vi "saveUserAnd SystemConfigFiles.vi"(10 "controls":T1 {"allValues"."safetyLimits"."channelLimits"."channelID" items=["time", "gearbox", "compressor bearing", "shaft bearing", "oil outlet", "inlet 1", "inlet 2", "outlet 1", "outlet 2", "inlet pressure", "outlet pressure", "plenum pressure", "Motor speed", "new V-cone DP", "Motor power", "Accelerometer", "Hotwire 1", "oil pressure", "butterfly valve position", "ball valve position", "Legacy speed", "Torque speed", "pulsator encoder", "v-cone upstream 1", "v-cone upstream 2"]}) -> ()   [LabVIEW 2018]
uses:
  user interface/systemConfigUIControls.ctl
  type defs/channelLimitControl.ctl
  type defs/limitActions.ctl
  ICL-LabVIEW_General/data channels/parent class/Data Channel.lvclass
  RT/Type Defs/Message loop data.ctl
  RT/Type Defs/FPGA reference.ctl
  RT/Type Defs/RT Status.ctl
  RT/Type Defs/Analogue loop data.ctl
  RT/Communications loop/comms data.ctl
  RT/Type Defs/generic incident.ctl
  ICL-LabVIEW_General/Scanivalve API project/full interface/polymorphic/scanivalveConfig.ctl
  ICL-LabVIEW_General/Scanivalve API project/full interface/listS.ctl
  ICL-LabVIEW_General/Scanivalve API project/full interface/listC.ctl
  ICL-LabVIEW_General/Scanivalve API project/full interface/listSG.ctl
  ICL-LabVIEW_General/Scanivalve API project/full interface/chan1.ctl
  RT/Type Defs/Data processing loop data.ctl
  type defs/channelControl.ctl
  RT/Type Defs/channelScalingTypes.ctl
  RT/Type Defs/scalingMethods.ctl
  <vilib>/Utility/config.llb/Write Key (String).vi
  <vilib>/Utility/config.llb/Write Key (Path).vi
  <vilib>/Utility/config.llb/Write Key (U32).vi
  <vilib>/Utility/config.llb/Write Key (Boolean).vi
  <vilib>/Utility/config.llb/Write Key (Double).vi
  <vilib>/Utility/config.llb/NI_LVConfig.lvlib
  ICL-LabVIEW_General/data channels/data channels.lvlib
  ICL-LabVIEW_General/Scanivalve API project/Scanivalve API.lvlib
panel:
  out "error out":errorcluster
  out "unwritten keys":string[](array[string])
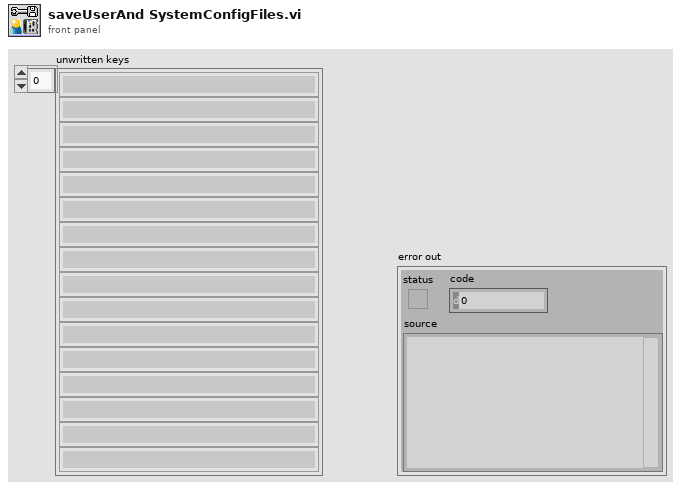
[diagram p1: front panel]
types:
  T1 = typedef "systemConfigUIControls.ctl" = cluster{"allControls":cluster{"feedbackChannels":cluster{"butterfly":refnum<vi>, "ball":refnum<vi>, "massflow":refnum<vi>, "pressureRatio":refnum<vi>, "airP":refnum<vi>, "water":refnum<vi>, "oilP":refnum<vi>, "speed":refnum<vi>}, "controlChannels":cluster{"butterflyControl":refnum<vi>, "ballControl":refnum<vi>, "speedControl":refnum<vi>}, "channelLimits":refnum<vi>, "pulsatorIP":string}, "allValues":cluster{"feedback":cluster{"butterfly":u16, "ball":u16, "massflow":u16, "pressureRatio":u16, "airP":u16, "water":u16, "oilP":u16, "speed":u16}, "paths":cluster{"channelConfig":path, "systemConfig":path, "incidentLogfile":path, "startFolder":path, "customVI":path}, "RT":cluster{"RTIP":string, "errorReaderName":string, "errorWriterName":string, "errorBufferSize":u16, "commandWriterName":string, "commandReaderName":string, "commandBufferSize":u16, "dataBufferSize":u16, "dataReaderName":string, "dataWriterName":string, "dataBufferLength":u16, "scanivalveIP":string, "scanPeriod":u16}, "controls":cluster{"butterflyControl":u16, "ballControl":u16, "speedControl":u16}, "safetyLimits":cluster{"channelLimits":T2[], "maxSpeed":u32}, "Howden":cluster{"howdenAir":bool, "howden%":dbl}}, "variables":cluster{"feedbackChannelIDs":u16[], "controlChannelIDs":u16[], "channelsArray":refnum<class "Data Channel.lvclass">[]}}
  T2 = typedef "channelLimitControl.ctl" = cluster{"channelID":u16, "Enabled":bool, "warnValue":dbl, "limitValue":dbl, "Invert":bool, "limitAction":T3}
  T3 = typedef "limitActions.ctl" = enum16{"stop", "shutdown", "ignore"}
  T4 = typedef "Message loop data.ctl" = cluster{"Parameters":cluster{"FPGA Ref":T5, "configID":u32, "activeChannels":cluster{"index":u16, "name":string}[]}, "Variables":cluster{"RT Status":T6, "watchdog":timestamp, "limitsEnabled":bool, "Interlocks":cluster{"gearboxOil":bool, "bearingOil":bool, "gearboxAir":bool}}}
  T5 = typedef "FPGA reference.ctl" = refnum<k20>
  T6 = typedef "RT Status.ctl" = cluster{"Comms loop":bool, "scheduler loop":bool, "data process loop":bool, "FIFO loop":bool, "Command Stream":bool, "Error Stream":bool, "FPGA FIFO":bool, "Data Stream":bool}
  T7 = typedef "Analogue loop data.ctl" = cluster{"Params":cluster{"FPGA ref":T5, "Total Channels":u32}, "Variables":cluster{"FIFO wait counter":u16, "FIFO read trigger":u32}}
  T8 = typedef "comms data.ctl" = cluster{"Parameters":cluster{"error writer name":string, "command reader name":string, "error buffer size":i32, "command buffer size":i32, "scanivalveIP":string, "scanivalvePeriod":u16}, "Variables":cluster{"listen schedule":u32, "incident buffer":T9[], "command stream":refnum<k21>, "error stream":refnum<k21>, "waiting for command stream connect":bool, "waiting for error stream connect":bool, "scanivalve connection":refnum<k5>, "scanivalveScheduleID":u32, "activeScanivalvePorts":i32[], "channelCount":i16}, "scanivalveConfig":T10}
  T9 = typedef "generic incident.ctl" = cluster{"timestamp":timestamp, "type":string, "Variant":variant}
  T10 = typedef "Scanivalve API.lvlib/scanivalveConfig.ctl" = cluster{"listS":T11, "listC":T12, "listSG":T13, "activeChannels":T14}
  T11 = typedef "Scanivalve API.lvlib/listS.ctl" = cluster{"period":u16, "ADtrig":bool, "ScanTrig":bool, "page":u16, "qpkts":u16}
  T12 = typedef "Scanivalve API.lvlib/listC.ctl" = cluster{"ZC":bool, "unitScan":string, "CvtUnit":dbl, "bin":bool, "EU":bool}
  T13 = typedef "Scanivalve API.lvlib/listSG.ctl" = cluster{"Avg1":u16, "FPS1":u16, "SGEnable1":bool}
  T14 = typedef "Scanivalve API.lvlib/chan1.ctl" = cluster{"Chan1":cluster{"101":bool, "102":bool, "103":bool, "104":bool, "109":bool, "110":bool, "111":bool, "112":bool, "201":bool, "202":bool, "203":bool, "204":bool, "209":bool, "210":bool, "211":bool, "212":bool, "301":bool, "302":bool, "303":bool, "304":bool, "309":bool, "310":bool, "311":bool, "312":bool, "401":bool, "402":bool, "403":bool, "404":bool, "409":bool, "410":bool, "411":bool, "412":bool}}
  T15 = typedef "Data processing loop data.ctl" = cluster{"Parameters":cluster{"FPGA Ref":T5, "data stream":cluster{"data writer name":string, "NS write buffer size":i32, "NS Buffer length":u32}, "FIFO Depth":u32, "Channel controls":cluster{"FIFO channel count":i32, "active indices":i16[], "active channels":i32, "channelScaling":T16[], "scanivalveCount":i32, "channels":refnum<class "Data Channel.lvclass">[]}, "safetyChannels":cluster{"oilP":u16, "airP":u16, "water":u16, "channelLimits":T2[]}, "speedChannel":i32, "maxSpeedLimit":dbl, "Torque":cluster{"fixedOffset":dbl, "filter":bool, "fallingEdge":bool, "swapEncoders":bool}}, "Variables":cluster{"Intermediary buffer":dbl[][], "buffer position":u32, "write loop counter":u16, "NS write trigger":u32, "NS Connection status":bool, "waiting for NS":bool, "labAmbient":cluster{"pressure":dbl, "temperature":dbl}, "scanivalvePorts":u16[], "scanivalvePressures":dbl[], "data stream":refnum<k21>, "activeChannelLimitIndex":u16[], "runningSpeedLimit":dbl, "speedChannelIndex":i32, "Interlocks":cluster{"gearboxOil":bool, "bearingOil":bool, "gearboxAir":bool}, "interlockChannels":cluster{"gearboxOil":i32, "bearingOil":i32, "air":i32}, "limitStates":cluster{"warn":bool, "alarm":bool}[]}}
  T16 = typedef "channelControl.ctl" = cluster{"index":u16, "active":bool, "channelType":T17, "module":u16, "terminal":u16, "channelName":string, "scalingMethod":T18, "scalingParameters":dbl[], "scaledUnits":string, "tempOffset":dbl}
  T17 = typedef "channelScalingTypes.ctl" = enum16{"calculation", "measurement", "scanivalve", "output", "digital"}
  T18 = typedef "scalingMethods.ctl" = enum16{"none", "linear", "thermocouple", "polynomial", "encoder", "RTD"}
  T19 = cluster{"Message":T4, "FIFO":T7, "Comms data":T8, "Data processor":T15}
  T20 = cluster{"total":cluster{"channels":u16, "FIFO":u16, "Scanivalve":u16, "Remote":u16, "Calculated":u16}, "active":cluster{"channels":u16, "FIFO":u16, "Scanivalve":u16, "Remote":u16, "Calculated":u16}}
  T21 = typedef "NI_LVConfig.lvlib/Config Data RefNum.ctl" = refnum<k1>
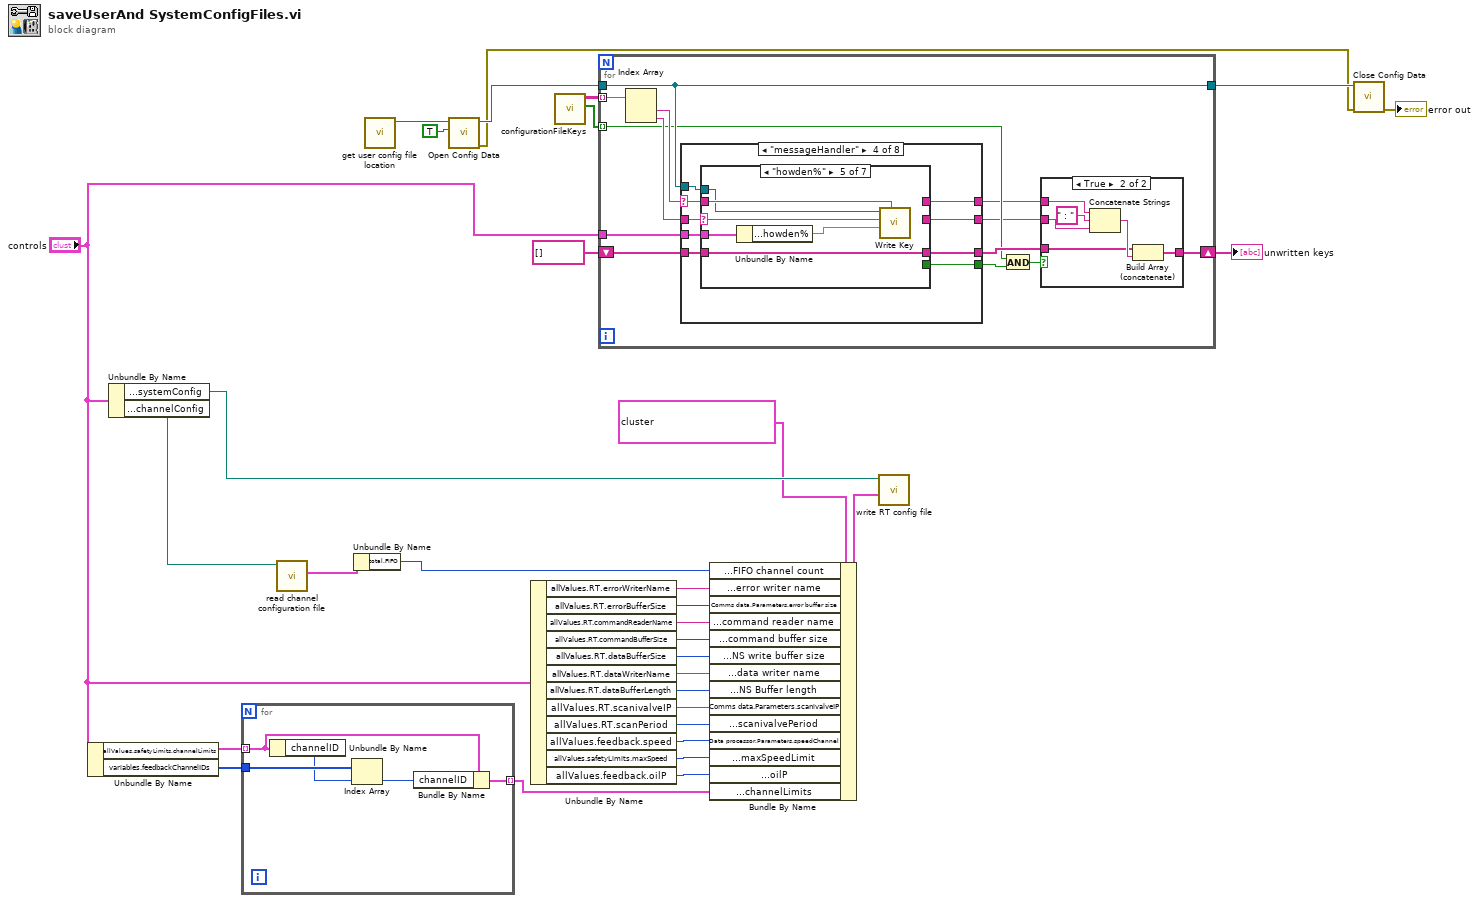
[diagram p0: block diagram]
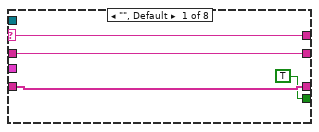
[diagram p3: hidden frame]
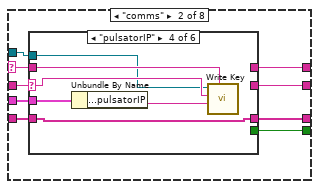
[diagram p4: hidden frame]
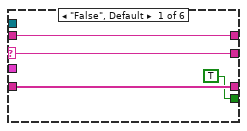
[diagram p5: hidden frame]
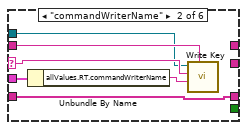
[diagram p6: hidden frame]
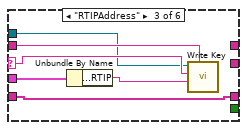
[diagram p7: hidden frame]
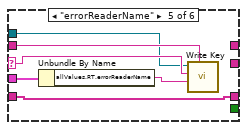
[diagram p8: hidden frame]
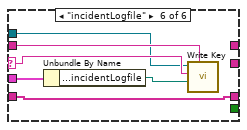
[diagram p9: hidden frame]
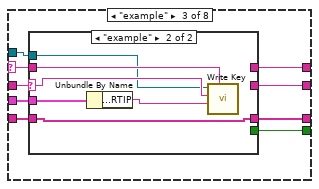
[diagram p10: hidden frame]
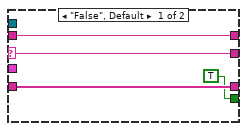
[diagram p11: hidden frame]
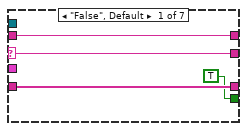
[diagram p12: hidden frame]
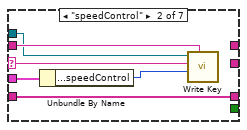
[diagram p13: hidden frame]
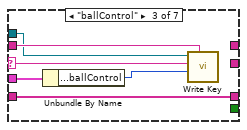
[diagram p14: hidden frame]
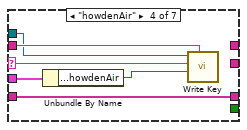
[diagram p15: hidden frame]
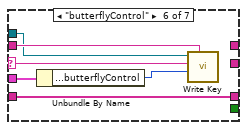
[diagram p16: hidden frame]
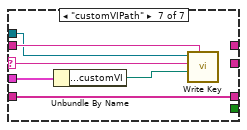
[diagram p17: hidden frame]
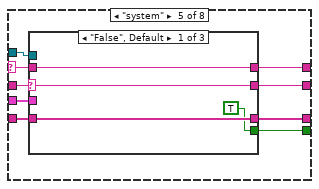
[diagram p18: hidden frame]
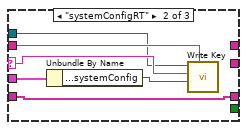
[diagram p19: hidden frame]
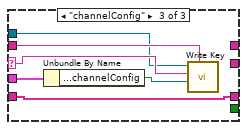
[diagram p20: hidden frame]
diagram:
  n1 = Unbundle By Name("controls") -> ("allValues.safetyLimits.channelLimits"=w10:T2[], "variables.feedbackChannelIDs"=w9:u16[])
  n2 = Unbundle By Name("controls") -> ("allValues.paths.systemConfig"=w22:path, "allValues.paths.channelConfig"=w5:path)
  n3 = for {
    tunnel: w10 -> [w34] mode=indexing
    tunnel: w9 -> [w37]
    tunnel: [w33] -> w1 mode=indexing
    n4 = Unbundle By Name(w34) -> ("channelID"=w36:u16)
    n5 = Index Array(array=w37, index=w36) -> (element=w35:u16)
    n6 = Bundle By Name(cluster=w34, "channelID"=w35) -> (w33:T2)
  }
  n7 = call "read channel configuration file.vi"("config file"=w5) -> ("counts"=w4:T20)  [unwired: 8 in, 2 out]
  n8 = Unbundle By Name(w4) -> ("total.FIFO"=w3:u16)
  n9 = call "get user config file location.vi"() -> ("userConfigPath"=w31:path)  [unwired: 11 in]
  n10 = call <vilib>:"Open Config Data.vi"("create file if necessary (T)"=TRUE, "configuration file path"=w31) -> ("error out"=w23:errorcluster, "refnum"=w30:T21)  [unwired: 7 in, 1 out]
  n11 = Unbundle By Name("controls") -> ("allValues.RT.errorWriterName"=w19:string, "allValues.RT.errorBufferSize"=w18:u16, "allValues.RT.commandReaderName"=w17:string, "allValues.RT.commandBufferSize"=w16:u16, "allValues.RT.dataBufferSize"=w15:u16, "allValues.RT.dataWriterName"=w14:string, "allValues.RT.dataBufferLength"=w13:u16, "allValues.RT.scanivalveIP"=w12:string, "allValues.RT.scanPeriod"=w11:u16, "allValues.feedback.speed"=w8:u16, "allValues.safetyLimits.maxSpeed"=w6:u32, "allValues.feedback.oilP"=w2:u16)
  n12 = call "configurationFileKeys.vi"() -> ("write user key?"=w25:bool[], "userConfigKeys"=w32:string[][])  [unwired: 9 in, 1 out]
  n13 = for {
    tunnel: "controls" -> [w46]
    tunnel: w32 -> [w50] mode=indexing
    tunnel: w30 -> [w47]
    tunnel: [w47] -> w29
    shift-right: [w43] -> w26
    shift-left: string[] [] -> [w45]
    tunnel: w25 -> [w41] mode=indexing
    n14 = Index Array(array=w50) -> (element #1=w49:string, element #2=w48:string)  [unwired: 2 in]
    n15 = case shown="\"messageHandler\"" w49 {
      selector: w49 -> [w61 w67 w110 w129 w178 w203 w252 w271]
      tunnel: w48 -> [w60 w70 w113 w132 w181 w206 w255 w274]
      tunnel: w47 -> [_ w69 w112 w131 w180 w205 w254 w273]
      tunnel: w46 -> [_ w68 w111 w130 w179 w204 w253 w272]
      tunnel: [w59 w66 w109 w128 w177 w202 w251 w270] -> w44
      tunnel: w45 -> [w59 w65 w108 w127 w176 w201 w250 w269]
      tunnel: [TRUE w62 w105 w124 w175 w198 w247 w266] -> w42
      tunnel: [w61 w64 w107 w126 w174 w200 w249 w268] -> w39
      tunnel: [w60 w63 w106 w125 w173 w199 w248 w267] -> w38
      frame "", Default {
      }
      frame "comms" {
        n16 = case shown="\"pulsatorIP\"" w70 {
          selector: w70 -> [w72 w79 w85 w91 w97 w103]
          tunnel: w69 -> [_ w78 w84 w90 w96 w102]
          tunnel: w68 -> [_ w77 w83 w89 w95 w101]
          tunnel: w67 -> [w73 w80 w86 w92 w98 w104]
          tunnel: [w74 w75 w81 w87 w93 w99] -> w66
          tunnel: w65 -> [w74 w75 w81 w87 w93 w99]
          tunnel: [w73 _ _ _ _ _] -> w64
          tunnel: [w72 _ _ _ _ _] -> w63
          tunnel: [TRUE _ _ _ _ _] -> w62
          frame "False", Default {
          }
          frame "commandWriterName" {
            n17 = Unbundle By Name(w77) -> ("allValues.RT.commandWriterName"=w76:string)
            n18 = call-poly <vilib>:"Write Key.vi"("section"=w80, "value"=w76, "key"=w79, "refnum"=w78) -> ()  [unwired: 5 in, 3 out]
          }
          frame "RTIPAddress" {
            n19 = Unbundle By Name(w83) -> ("allValues.RT.RTIP"=w82:string)
            n20 = call-poly <vilib>:"Write Key.vi"("section"=w86, "value"=w82, "key"=w85, "refnum"=w84) -> ()  [unwired: 5 in, 3 out]
          }
          frame "pulsatorIP" {
            n21 = Unbundle By Name(w89) -> ("allControls.pulsatorIP"=w88:string)
            n22 = call-poly <vilib>:"Write Key.vi"("section"=w92, "value"=w88, "key"=w91, "refnum"=w90) -> ()  [unwired: 5 in, 3 out]
          }
          frame "errorReaderName" {
            n23 = Unbundle By Name(w95) -> ("allValues.RT.errorReaderName"=w94:string)
            n24 = call-poly <vilib>:"Write Key.vi"("section"=w98, "value"=w94, "key"=w97, "refnum"=w96) -> ()  [unwired: 5 in, 3 out]
          }
          frame "incidentLogfile" {
            n25 = Unbundle By Name(w101) -> ("allValues.paths.incidentLogfile"=w100:path)
            n26 = call-poly <vilib>:"Write Key.vi"("section"=w104, "value"=w100, "key"=w103, "refnum"=w102) -> ()  [unwired: 5 in, 3 out]
          }
        }
      }
      frame "example" {
        n27 = case shown="\"example\"" w113 {
          selector: w113 -> [w115 w122]
          tunnel: w112 -> [_ w121]
          tunnel: w111 -> [_ w120]
          tunnel: w110 -> [w116 w123]
          tunnel: [w117 w118] -> w109
          tunnel: w108 -> [w117 w118]
          tunnel: [w116 _] -> w107
          tunnel: [w115 _] -> w106
          tunnel: [TRUE _] -> w105
          frame "False", Default {
          }
          frame "example" {
            n28 = Unbundle By Name(w120) -> ("allValues.RT.RTIP"=w119:string)
            n29 = call-poly <vilib>:"Write Key.vi"("section"=w123, "value"=w119, "key"=w122, "refnum"=w121) -> ()  [unwired: 5 in, 3 out]
          }
        }
      }
      frame "messageHandler" {
        n30 = case shown="\"howden%\"" w132 {
          selector: w132 -> [w134 w141 w147 w153 w159 w165 w171]
          tunnel: w131 -> [_ w140 w146 w152 w158 w164 w170]
          tunnel: w130 -> [_ w139 w145 w151 w157 w163 w169]
          tunnel: w129 -> [w135 w142 w148 w154 w160 w166 w172]
          tunnel: [w136 w137 w143 w149 w155 w161 w167] -> w128
          tunnel: w127 -> [w136 w137 w143 w149 w155 w161 w167]
          tunnel: [w135 _ _ _ _ _ _] -> w126
          tunnel: [w134 _ _ _ _ _ _] -> w125
          tunnel: [TRUE _ _ _ _ _ _] -> w124
          frame "False", Default {
          }
          frame "speedControl" {
            n31 = Unbundle By Name(w139) -> ("allValues.controls.speedControl"=w138:u16)
            n32 = call-poly <vilib>:"Write Key.vi"("section"=w142, "value"=w138, "key"=w141, "refnum"=w140) -> ()  [unwired: 5 in, 3 out]
          }
          frame "ballControl" {
            n33 = Unbundle By Name(w145) -> ("allValues.controls.ballControl"=w144:u16)
            n34 = call-poly <vilib>:"Write Key.vi"("section"=w148, "value"=w144, "key"=w147, "refnum"=w146) -> ()  [unwired: 5 in, 3 out]
          }
          frame "howdenAir" {
            n35 = Unbundle By Name(w151) -> ("allValues.Howden.howdenAir"=w150:bool)
            n36 = call-poly <vilib>:"Write Key.vi"("section"=w154, "value"=w150, "key"=w153, "refnum"=w152) -> ()  [unwired: 5 in, 3 out]
          }
          frame "howden%" {
            n37 = Unbundle By Name(w157) -> ("allValues.Howden.howden%"=w156:dbl)
            n38 = call-poly <vilib>:"Write Key.vi"("section"=w160, "value"=w156, "key"=w159, "refnum"=w158) -> ()  [unwired: 5 in, 3 out]
          }
          frame "butterflyControl" {
            n39 = Unbundle By Name(w163) -> ("allValues.controls.butterflyControl"=w162:u16)
            n40 = call-poly <vilib>:"Write Key.vi"("section"=w166, "value"=w162, "key"=w165, "refnum"=w164) -> ()  [unwired: 5 in, 3 out]
          }
          frame "customVIPath" {
            n41 = Unbundle By Name(w169) -> ("allValues.paths.customVI"=w168:path)
            n42 = call-poly <vilib>:"Write Key.vi"("section"=w172, "value"=w168, "key"=w171, "refnum"=w170) -> ()  [unwired: 5 in, 3 out]
          }
        }
      }
      frame "system" {
        n43 = case shown="\"False\", Default" w181 {
          selector: w181 -> [w182 w190 w196]
          tunnel: w180 -> [_ w189 w195]
          tunnel: w179 -> [_ w188 w194]
          tunnel: w178 -> [w183 w191 w197]
          tunnel: [w185 w186 w192] -> w177
          tunnel: w176 -> [w185 w186 w192]
          tunnel: [TRUE _ _] -> w175
          tunnel: [w183 _ _] -> w174
          tunnel: [w182 _ _] -> w173
          frame "False", Default {
          }
          frame "systemConfigRT" {
            n44 = Unbundle By Name(w188) -> ("allValues.paths.systemConfig"=w187:path)
            n45 = call-poly <vilib>:"Write Key.vi"("section"=w191, "value"=w187, "key"=w190, "refnum"=w189) -> ()  [unwired: 5 in, 3 out]
          }
          frame "channelConfig" {
            n46 = Unbundle By Name(w194) -> ("allValues.paths.channelConfig"=w193:path)
            n47 = call-poly <vilib>:"Write Key.vi"("section"=w197, "value"=w193, "key"=w196, "refnum"=w195) -> ()  [unwired: 5 in, 3 out]
          }
        }
      }
      frame "dataProcessor" {
        n48 = case shown="\"oilPressure\"" w206 {
          selector: w206 -> [w208 w215 w221 w227 w233 w239 w245]
          tunnel: w205 -> [_ w214 w220 w226 w232 w238 w244]
          tunnel: w204 -> [_ w213 w219 w225 w231 w237 w243]
          tunnel: w203 -> [w209 w216 w222 w228 w234 w240 w246]
          tunnel: [w210 w211 w217 w223 w229 w235 w242] -> w202
          tunnel: w201 -> [w210 w211 w217 w223 w229 w235 w242]
          tunnel: [w209 _ _ _ _ _ _] -> w200
          tunnel: [w208 _ _ _ _ _ _] -> w199
          tunnel: [TRUE _ _ _ _ _ _] -> w198
          frame "False", Default {
          }
          frame "speedChannel" {
            n49 = Unbundle By Name(w213) -> ("allValues.feedback.speed"=w212:u16)
            n50 = call-poly <vilib>:"Write Key.vi"("section"=w216, "value"=w212, "key"=w215, "refnum"=w214) -> ()  [unwired: 5 in, 3 out]
          }
          frame "oilPressure" {
            n51 = Unbundle By Name(w219) -> ("allValues.feedback.oilP"=w218:u16)
            n52 = call-poly <vilib>:"Write Key.vi"("section"=w222, "value"=w218, "key"=w221, "refnum"=w220) -> ()  [unwired: 5 in, 3 out]
          }
          frame "butterflyChannel" {
            n53 = Unbundle By Name(w225) -> ("allValues.feedback.butterfly"=w224:u16)
            n54 = call-poly <vilib>:"Write Key.vi"("section"=w228, "value"=w224, "key"=w227, "refnum"=w226) -> ()  [unwired: 5 in, 3 out]
          }
          frame "ballChannel" {
            n55 = Unbundle By Name(w231) -> ("allValues.feedback.ball"=w230:u16)
            n56 = call-poly <vilib>:"Write Key.vi"("section"=w234, "value"=w230, "key"=w233, "refnum"=w232) -> ()  [unwired: 5 in, 3 out]
          }
          frame "massflow" {
            n57 = Unbundle By Name(w237) -> ("allValues.feedback.massflow"=w236:u16)
            n58 = call-poly <vilib>:"Write Key.vi"("section"=w240, "value"=w236, "key"=w239, "refnum"=w238) -> ()  [unwired: 5 in, 3 out]
          }
          frame "pressureRatio" {
            n59 = Unbundle By Name(w243) -> ("allValues.feedback.pressureRatio"=w241:u16)
            n60 = call-poly <vilib>:"Write Key.vi"("section"=w246, "value"=w241, "key"=w245, "refnum"=w244) -> ()  [unwired: 5 in, 3 out]
          }
        }
      }
      frame "fileIO" {
        n61 = case shown="\"False\", Default" w255 {
          selector: w255 -> [w257 w264]
          tunnel: w254 -> [_ w263]
          tunnel: w253 -> [_ w262]
          tunnel: w252 -> [w258 w265]
          tunnel: [w259 w260] -> w251
          tunnel: w250 -> [w259 w260]
          tunnel: [w258 _] -> w249
          tunnel: [w257 _] -> w248
          tunnel: [TRUE _] -> w247
          frame "False", Default {
          }
          frame "startFolder" {
            n62 = Unbundle By Name(w262) -> ("allValues.paths.startFolder"=w261:path)
            n63 = call-poly <vilib>:"Write Key.vi"("section"=w265, "value"=w261, "key"=w264, "refnum"=w263) -> ()  [unwired: 5 in, 3 out]
          }
        }
      }
      frame "dataStream" {
        n64 = case shown="\"False\", Default" w274 {
          selector: w274 -> [w276 w283]
          tunnel: w273 -> [_ w282]
          tunnel: w272 -> [_ w281]
          tunnel: w271 -> [w277 w284]
          tunnel: [w278 w279] -> w270
          tunnel: w269 -> [w278 w279]
          tunnel: [w277 _] -> w268
          tunnel: [w276 _] -> w267
          tunnel: [TRUE _] -> w266
          frame "False", Default {
          }
          frame "dataReaderName" {
            n65 = Unbundle By Name(w281) -> ("allValues.RT.dataReaderName"=w280:string)
            n66 = call-poly <vilib>:"Write Key.vi"("section"=w284, "value"=w280, "key"=w283, "refnum"=w282) -> ()  [unwired: 5 in, 3 out]
          }
        }
      }
    }
    n67 = And(x=w41, y=w42) -> (x .and. y?=w40:bool)
    n68 = case shown="True" w40 {
      tunnel: [w51 w54] -> w43
      tunnel: w44 -> [w51 w55]
      tunnel: w39 -> [_ w53]
      tunnel: w38 -> [_ w52]
      frame False {
      }
      frame True {
        n69 = Concatenate Strings(w53, " : " ("string"), w52) -> (w56:string)
        n70 = Build Array (concatenate)(w55, w56) -> (w54:string[])
      }
    }
  }
  "unwritten keys" <- w26
  n71 = Bundle By Name(cluster=T19 {"Message"={"Parameters"={"FPGA Ref"=refnum, "configID"=0, "activeChannels"=[]}, "Variables"={"RT Status"={"Comms loop"=FALSE, "scheduler loop"=FALSE, "data process loop"=FALSE, "FIFO loop"=FALSE, "Command Stream"=FALSE, "Error Stream"=FALSE, "FPGA FIFO"=FALSE, "Data Stream"=FALSE}, "watchdog"=timestamp(0 s since 1904-01-01), "limitsEnabled"=FALSE, "Interlocks"={"gearboxOil"=FALSE, "bearingOil"=FALSE, "gearboxAir"=FALSE}}}, "FIFO"={"Params"={"FPGA ref"=refnum, "Total Channels"=0}, "Variables"={"FIFO wait counter"=0, "FIFO read trigger"=0}}, "Comms data"={"Parameters"={"error writer name"="errorWriter", "command reader name"="commandReader", "error buffer size"=16, "command buffer size"=10, "scanivalveIP"="155.198.87.12", "scanivalvePeriod"=500}, "Variables"={"listen schedule"=0, "incident buffer"=[], "command stream"="", "error stream"="", "waiting for command stream connect"=FALSE, "waiting for error stream connect"=FALSE, "scanivalve connection"=refnum, "scanivalveScheduleID"=16, "activeScanivalvePorts"=[], "channelCount"=0}, "scanivalveConfig"={"listS"={"period"=0, "ADtrig"=FALSE, "ScanTrig"=FALSE, "page"=0, "qpkts"=0}, "listC"={"ZC"=FALSE, "unitScan"="", "CvtUnit"=0.0, "bin"=FALSE, "EU"=FALSE}, "listSG"={"Avg1"=0, "FPS1"=0, "SGEnable1"=FALSE}, "activeChannels"={"Chan1"={"101"=FALSE, "102"=FALSE, "103"=FALSE, "104"=FALSE, "109"=FALSE, "110"=FALSE, "111"=FALSE, "112"=FALSE, "201"=FALSE, "202"=FALSE, "203"=FALSE, "204"=FALSE, "209"=FALSE, "210"=FALSE, "211"=FALSE, "212"=FALSE, "301"=FALSE, "302"=FALSE, "303"=FALSE, "304"=FALSE, "309"=FALSE, "310"=FALSE, "311"=FALSE, "312"=FALSE, "401"=FALSE, "402"=FALSE, "403"=FALSE, "404"=FALSE, "409"=FALSE, "410"=FALSE, "411"=FALSE, "412"=FALSE}}}}, "Data processor"={"Parameters"={"FPGA Ref"=refnum, "data stream"={"data writer name"="", "NS write buffer size"=0, "NS Buffer length"=0}, "FIFO Depth"=0, "Channel controls"={"FIFO channel count"=0, "active indices"=[], "active channels"=0, "channelScaling"=[], "scanivalveCount"=0, "channels"=[]}, "safetyChannels"={"oilP"=0, "airP"=0, "water"=0, "channelLimits"=[]}, "speedChannel"=0, "maxSpeedLimit"=0.0, "Torque"={"fixedOffset"=0.0, "filter"=FALSE, "fallingEdge"=FALSE, "swapEncoders"=FALSE}}, "Variables"={"Intermediary buffer"=[], "buffer position"=0, "write loop counter"=0, "NS write trigger"=0, "NS Connection status"=FALSE, "waiting for NS"=FALSE, "labAmbient"={"pressure"=0.0, "temperature"=0.0}, "scanivalvePorts"=[], "scanivalvePressures"=[], "data stream"="", "activeChannelLimitIndex"=[], "runningSpeedLimit"=0.0, "speedChannelIndex"=0, "Interlocks"={"gearboxOil"=FALSE, "bearingOil"=FALSE, "gearboxAir"=FALSE}, "interlockChannels"={"gearboxOil"=0, "bearingOil"=0, "air"=0}, "limitStates"=[]}}} ("RT config"), "Data processor.Parameters.Channel controls.FIFO channel count"=w3, "Comms data.Parameters.error writer name"=w19, "Comms data.Parameters.error buffer size"=w18, "Comms data.Parameters.command reader name"=w17, "Comms data.Parameters.command buffer size"=w16, "Data processor.Parameters.data stream.NS write buffer size"=w15, "Data processor.Parameters.data stream.data writer name"=w14, "Data processor.Parameters.data stream.NS Buffer length"=w13, "Comms data.Parameters.scanivalveIP"=w12, "Comms data.Parameters.scanivalvePeriod"=w11, "Data processor.Parameters.speedChannel"=w8, "Data processor.Parameters.maxSpeedLimit"=w6, "Data processor.Parameters.safetyChannels.oilP"=w2, "Data processor.Parameters.safetyChannels.channelLimits"=w1) -> (w20:T19)
  n72 = call "write RT config file.vi"("RT config"=w20, "RT config file path"=w22) -> ()  [unwired: 10 in]
  n73 = call <vilib>:"Close Config Data.vi"("error in (no error)"=w23, "refnum"=w29) -> ("error out"=→"error out":errorcluster)  [unwired: 8 in, 1 out]
